vi "IntraX.vi"(8 "error in (no error)":errorcluster, 11 "Momentum [MeV/C](pixel)":dbl[](array[numeric])) -> (0 "error out":errorcluster, 1 "delta momentum":dbl, 2 "IntraX":i32, 3 "Ramp Pattern":dbl[](array[numeric]))   [LabVIEW 2020]
uses:
  <vilib>/Analysis/1siggen.llb/Ramp Pattern by Delta.vi
  <vilib>/Analysis/NI_AALBase.lvlib
panel:
  out "x/y":dbl
  out "Momentum [MeV/C](pixel) 2":dbl[](graph)
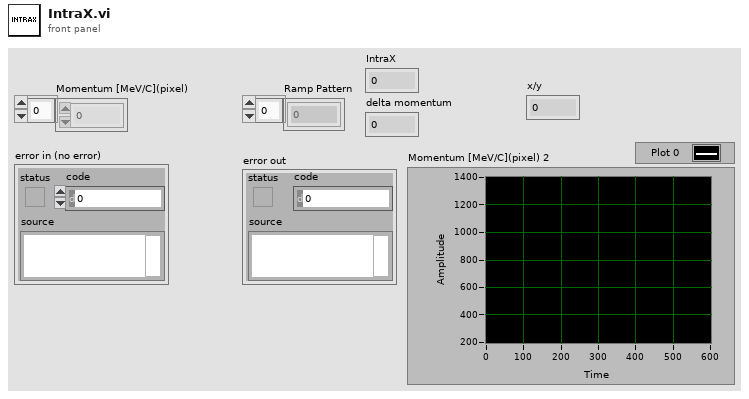
[diagram p1: front panel]
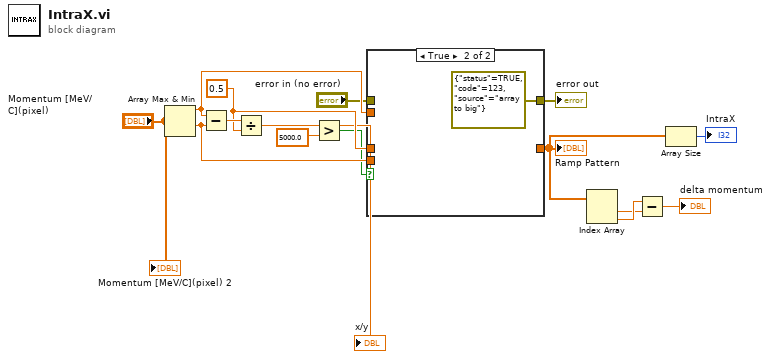
[diagram p0: block diagram]
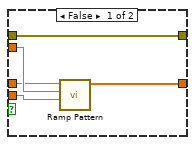
[diagram p2: hidden frame]
diagram:
  w11 = 0.5 ("delta")
  n1 = Array Max & Min(array="Momentum [MeV/C](pixel)") -> (max value=w14:dbl, min value=w13:dbl)  [unwired: 2 out]
  n2 = Subtract(x=w14, y=w13) -> (x-y=w12:dbl)
  n3 = Divide(x=w12, y=w11) -> (x/y=w10:dbl)
  "x/y" <- w10
  n4 = Greater?(x=w10, y=5000.0) -> (0:w8:bool)
  n5 = case shown="True" w8 {
    tunnel: [w20 _] -> w2
    tunnel: w14 -> [w19 _]
    tunnel: w13 -> [w18 _]
    tunnel: w11 -> [w17 _]
    tunnel: [w16 errorcluster {"status"=TRUE, "code"=123, "source"="array to big"} ("error in (no error)")] -> w7
    tunnel: "error in (no error)" -> [w16 _]
    frame False {
      n6 = call-poly <vilib>:"Ramp Pattern.vi"("start"=w18, "end"=w19, "delta"=w17) -> ("Ramp Pattern"=w20:dbl[])  [unwired: 6 in, 2 out]
    }
    frame True {
    }
  }
  "Ramp Pattern" <- w2
  "error out" <- w7
  n7 = Index Array(array=w2) -> (element #1=w3:dbl, element #2=w4:dbl)  [unwired: 2 in]
  n8 = Subtract(x=w4, y=w3) -> (x-y=→"delta momentum":dbl)
  n9 = Array Size(array=w2) -> (size(s)=→"IntraX":i32)
  "Momentum [MeV/C](pixel) 2" <- "Momentum [MeV/C](pixel)"
